vi "FM_Radio_Spectrum 1.vi"() -> ()   [LabVIEW 2016]
uses:
  <vilib>/measure/maspectr.llb/FFT Power Spectrum and PSD for 1 Chan (CDB).vi
  <instrlib>/niUSRP/niUSRP Fetch Rx Data (CDB WDT).vi
  <vilib>/measure/NI_MAPro.lvlib
panel:
  in  "Sound Format":T1={"channel"=enum."mono", "sample rate (S/s)"=enum."44100", "bits per sample"=enum."16 bit"}
  out "Frequency Spectrum":cluster{"f0":dbl, "df":dbl, "magnitude":dbl[]}(graph)={"f0"=-2500000.0, "df"=250.0, "magnitude"=[]}
  out "Time Domain Audio":waveform(dbl)(graph)={"t0"=timestamp(0 s since 1904-01-01), "dt"=2.2727272727272726e-05, "Y"=[]}
  in  "Stop":bool
  in  "number of samples":i64=20000
  in  "device names":refnum<k15>="192.168.10.2"
  in  "active antenna":string="RX2"
  in  "gain":dbl=25.0 format="%#_6f"
  in  "carrier frequency":dbl=105900000.0 format="%#_6p"
  in  "IQ rate":dbl=5000000.0 format="%#_6p"
  out "error out":errorcluster
  # "Broadcast FM Radio"
  # "NI USRP Configuration"
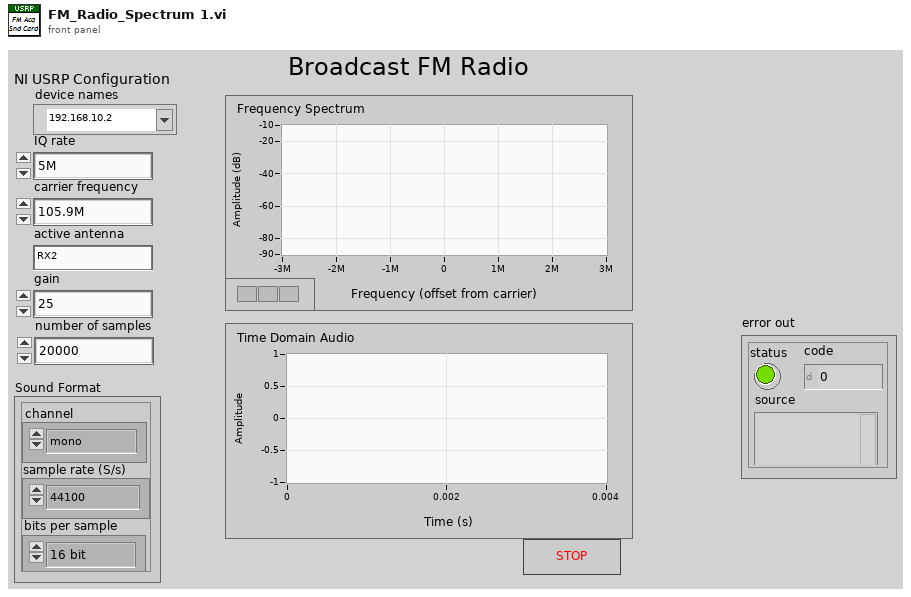
[diagram p1: front panel]
types:
  T1 = cluster{"channel":enum16{"mono", "stereo"}, "sample rate (S/s)":enum16{"11025", "22050", "44100", "8000"}, "bits per sample":enum16{"8 bit", "16 bit"}}
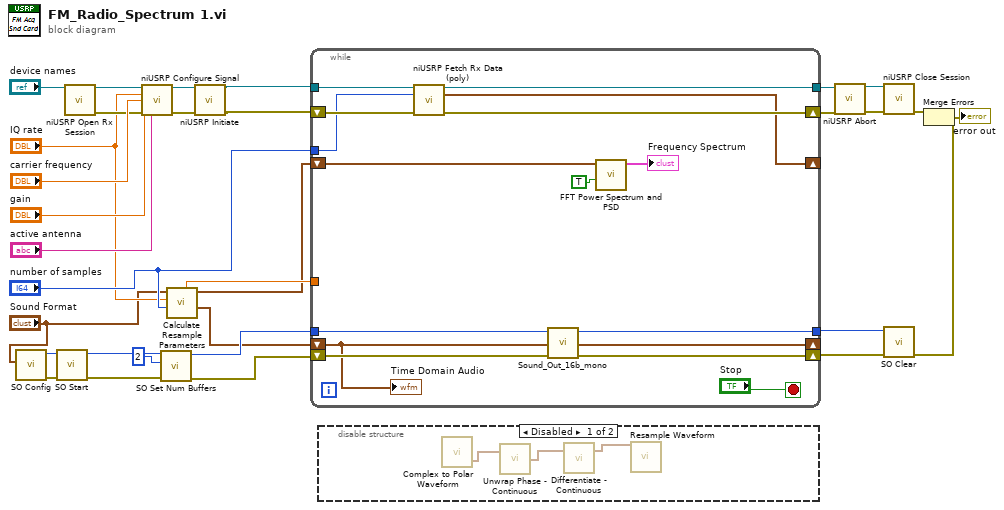
[diagram p0: block diagram]
diagram:
  n1 = call <vilib>:"SO Config.vi"("sound format"="Sound Format") -> ("error out"=w12:errorcluster, "task ID out"=w11:u32)  [unwired: 9 in]
  n2 = call <vilib>:"SO Start.vi"("error in (no error)"=w12, "task ID in"=w11) -> ("error out"=w8:errorcluster, "task ID out"=w9:u32)  [unwired: 8 in]
  n3 = call <instrlib>:"niUSRP Open Rx Session.vi"("device names"="device names") -> ("session handle out"=w32:refnum<k15>, "error out"=w30:errorcluster)  [unwired: 13 in]
  n4 = call <instrlib>:"niUSRP Configure Signal.vi"("session handle"=w32, "IQ rate"="IQ rate", "carrier frequency"="carrier frequency", "gain"="gain", "error in (no error)"=w30, "active antenna"="active antenna") -> ("session handle out"=w28:refnum<k15>, "error out"=w29:errorcluster)  [unwired: 5 in, 3 out]
  n5 = call <vilib>:"SO Set Num Buffers.vi"("error in (no error)"=w8, "number of buffers"=2, "task ID in"=w9) -> ("error out"=w6:errorcluster, "task ID out"=w7:u32)  [unwired: 7 in]
  n6 = call "Calculate Resample Parameters.vi"("Original Frame Size (Samples)"="number of samples", "Original Sample Rate (S/s)"="IQ rate", "Sound Format"="Sound Format") -> ("Audio Waveform Init"=w1:waveform(dbl), "IQ Waveform Init"=w15:waveform(cdb), "Resample Rate (dt)"=w16:dbl)  [unwired: 5 in, 1 out]
  n7 = call <instrlib>:"niUSRP Initiate.vi"("session handle"=w28, "error in (no error)"=w29) -> ("session handle out"=w14:refnum<k15>, "error out"=w13:errorcluster)  [unwired: 12 in]
  n8 = while {
    tunnel: w14 -> [w47]
    shift-right: [w44] -> w21
    shift-left: w13 -> [w46]
    tunnel: [w45] -> w22
    tunnel: "number of samples" -> [w42]
    shift-right: [w33] -> _
    shift-left: w1 -> [w33]
    shift-right: [w35] -> w4
    shift-left: w6 -> [w37]
    tunnel: [w36] -> w5
    shift-right: [w41] -> _
    shift-left: w15 -> [w34]
    tunnel: w16 -> [_]
    tunnel: w7 -> [w38]
    stop <- "Stop" stop-if-true
    n9 = call-poly <instrlib>:"niUSRP Fetch Rx Data (poly).vi"("session handle"=w47, "number of samples"=w42, "error in (no error)"=w46) -> ("session handle out"=w45:refnum<k15>, "data"=w41:waveform(cdb), "error out"=w44:errorcluster)  [unwired: 9 in, 1 out]
    n10 = call "Sound_Out_16b_mono.vi"("error in (no error)"=w37, "Audio Waveform Init"=w33, "task ID out in"=w38) -> ("error out"=w35:errorcluster, "task ID out out"=w36:u32)  [unwired: 7 in]
    n11 = call-poly <vilib>:"FFT Power Spectrum and PSD.vi"("dB On (F)"=TRUE, "time signal"=w34) -> ("Power Spectrum / PSD"=→"Frequency Spectrum":cluster{"f0":dbl, "df":dbl, "magnitude":dbl[]})  [unwired: 6 in, 3 out]
    "Time Domain Audio" <- w33
  }
  n12 = disable-structure shown="Disabled" {
    frame Disabled {
      n13 = call "Complex to Polar Waveform.vi"() -> ("Angle"=w48:waveform(dbl))  [unwired: 1 in, 1 out]
      n14 = call "Unwrap Phase - Continuous.vi"("Input Signal"=w48) -> ("Phase Unwrapped"=w49:waveform(dbl))  [unwired: 1 in]
      n15 = call "Differentiate - Continuous.vi"("Input Signal"=w49) -> ("dx/dt"=w50:waveform(dbl))  [unwired: 2 in]
      n16 = call "Resample Waveform.vi"("waveform in"=w50) -> ()  [unwired: 11 in, 4 out]
    }
    frame Enabled {
    }
  }
  n17 = call <instrlib>:"niUSRP Abort.vi"("session handle"=w22, "error in (no error)"=w21) -> ("session handle out"=w24:refnum<k15>, "error out"=w23:errorcluster)  [unwired: 12 in]
  n18 = call <instrlib>:"niUSRP Close Session.vi"("session handle"=w24, "error in (no error)"=w23) -> ("error out"=w20:errorcluster)  [unwired: 13 in]
  n19 = call <vilib>:"SO Clear.vi"("error in (no error)"=w4, "task ID in"=w5) -> ("error out"=w3:errorcluster)  [unwired: 9 in]
  n20 = Merge Errors(w20, w3) -> (→"error out":errorcluster)
